vi "Configure Control Mode.vi"(8 "error in (no error)":errorcluster, 10 "Mode  (0: Remote)":u16(ring) items=["Remote", "Local"], 11 "VISA resource name":refnum<visa-resource-name>) -> (0 "error out":errorcluster, 3 "VISA resource name out":refnum<visa-resource-name>)   [LabVIEW 2013, in "IT6900.lvlib"]
doc: "Select control mode is <b>remote</b> or <b>local</b>."
uses:
  <instrlib>/IT6900/IT6900.lvlib
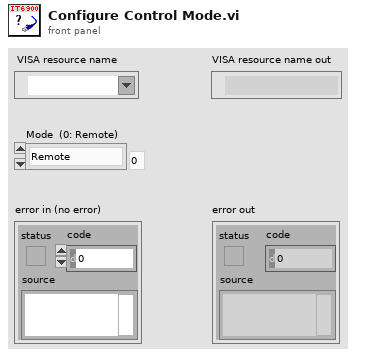
[diagram p1: front panel]
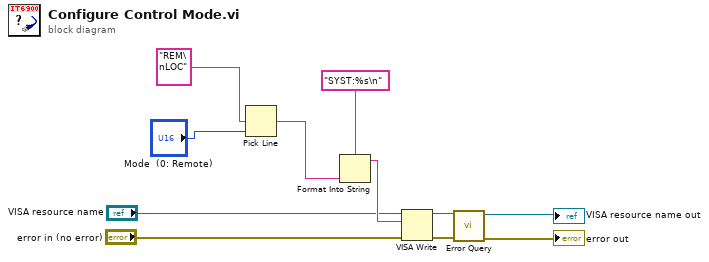
[diagram p0: block diagram]
diagram:
  n1 = Pick Line(multi-line string="REM\nLOC", line index="Mode  (0: Remote)") -> (output string=w9:string)  [unwired: 1 in]
  n2 = Format Into String(format string="SYST:%s\n", w9) -> (resulting string=w7:string)  [unwired: 2 in, 1 out]
  n3 = VISA Write(VISA resource name="VISA resource name", write buffer=w7, error in (no error)="error in (no error)") -> (VISA resource name out=w3:refnum<visa-resource-name>, error out=w4:errorcluster)  [unwired: 1 out]
  n4 = call <instrlib>:"Error Query.vi"("error in (no error)"=w4, "VISA resource name"=w3) -> ("error out"=→"error out":errorcluster, "VISA resource name out"=→"VISA resource name out":refnum<visa-resource-name>)  [unwired: 6 in, 2 out]
